vi "NamedRegAndResolve.vi"() -> ()   [LabVIEW 2024, in "Module Container.lvlib"]
uses:
  Module Container.lvlib
  Module/RQMHModule.lvclass
  Scripting/templates/TemplateModule/TemplateModule.lvclass
panel:
  out "Shouldn't Error":errorcluster
  out "Should Error":errorcluster
  in  "stop":bool
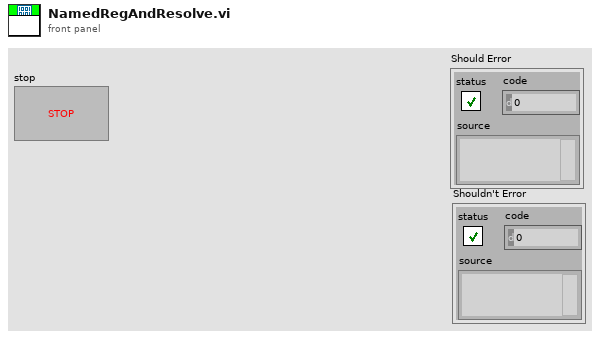
[diagram p1: front panel]
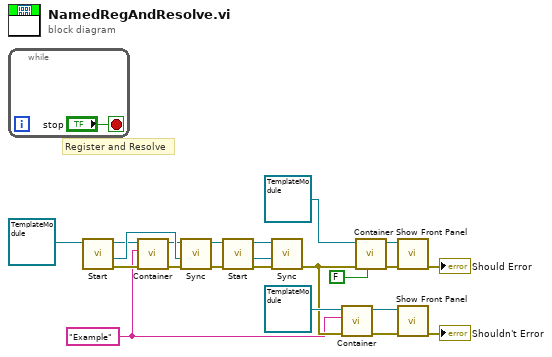
[diagram p0: block diagram]
diagram:
  w2 = "Example" ("Specific")
  # "Register and Resolve"
  n1 = while {
    stop <- "stop" stop-if-true
  }
  n2 = call "Start.vi"("JQMHCore in"=refnum<class "TemplateModule.lvclass"> refnum ("TemplateModule.lvclass")) -> ("error out"=w12:errorcluster, "StartupHandshake out"=w22:refnum<class "RQMHStartup.lvclass">, "JQMHCore out"=w16:refnum<class "TemplateModule.lvclass">)  [unwired: 8 in]
  n3 = call "Container.vi"("error in (no error)"=w12, "Specific"=w2, "Module Type"=w16) -> ("error out"=w11:errorcluster, "Module Instance"=w15:refnum<class "TemplateModule.lvclass">)  [unwired: 6 in, 1 out]
  n4 = call "Sync.vi"("error in (no error)"=w11, "StartupHandshake out"=w22, "JQMHCore in"=w15) -> ("error out"=w1:errorcluster, "JQMHCore out"=w19:refnum<class "TemplateModule.lvclass">)  [unwired: 7 in]
  n5 = call "Start.vi"("error in (no error)"=w1, "JQMHCore in"=w19) -> ("error out"=w20:errorcluster, "StartupHandshake out"=w17:refnum<class "RQMHStartup.lvclass">, "JQMHCore out"=w18:refnum<class "TemplateModule.lvclass">)  [unwired: 7 in]
  n6 = call "Sync.vi"("error in (no error)"=w20, "StartupHandshake out"=w17, "JQMHCore in"=w18) -> ("error out"=w6:errorcluster)  [unwired: 7 in, 1 out]
  n7 = call "Container.vi"("error in (no error)"=w6, "Specific"=w2, "Module Type"=refnum<class "TemplateModule.lvclass"> refnum ("TemplateModule.lvclass")) -> ("error out"=w5:errorcluster, "Module Instance"=w8:refnum<class "TemplateModule.lvclass">)  [unwired: 6 in, 1 out]
  n8 = call "Container.vi"("Start if not running? (T)"=FALSE, "error in (no error)"=w6, "Module Type"=refnum<class "TemplateModule.lvclass"> refnum ("TemplateModule.lvclass")) -> ("error out"=w4:errorcluster, "Module Instance"=w13:refnum<class "TemplateModule.lvclass">)  [unwired: 6 in, 1 out]
  n9 = call "Show Front Panel.vi"("error in (no error)"=w4, "JQMHCore in"=w13) -> ("error out"=→"Should Error":errorcluster)  [unwired: 8 in, 1 out]
  n10 = call "Show Front Panel.vi"("error in (no error)"=w5, "JQMHCore in"=w8) -> ("error out"=→"Shouldn't Error":errorcluster)  [unwired: 8 in, 1 out]
